vi "Derivative balance.vi"() -> (3 "Motor Power":dbl)   [LabVIEW 2020]
uses:
  Robot Global Data.vi
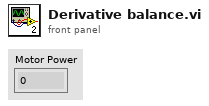
[diagram p1: front panel]
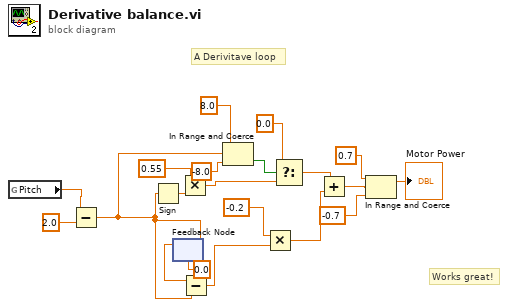
[diagram p0: block diagram]
diagram:
  # "Works great!"
  # "A Derivitave loop"
  n1 = global read "Robot Global Data.vi" "Pitch"() -> (w15:dbl)
  n2 = Subtract(x=w15, y=2.0) -> (x-y=w2:dbl)
  n3 = Sign(1:w2) -> (0:w5:dbl)
  n4 = feedback-in #1(w2) -> ()
  n5 = feedback #1(0.0) -> (w7:dbl)
  n6 = Multiply(x=0.55, y=w5) -> (x*y=w16:dbl)
  n7 = Subtract(x=w7, y=w2) -> (x-y=w19:dbl)
  n8 = In Range and Coerce(upper limit=8.0, x=w2, lower limit=-8.0) -> (In Range?=w12:bool)  [unwired: 1 out]
  n9 = Multiply(x=-0.2, y=w19) -> (x*y=w8:dbl)
  n10 = Select(t=0.0, s=w12, f=w16) -> (s? t:f=w10:dbl)
  n11 = Add(x=w10, y=w8) -> (x+y=w9:dbl)
  n12 = In Range and Coerce(upper limit=0.7, x=w9, lower limit=-0.7) -> (coerced(x)=→"Motor Power":dbl)  [unwired: 1 out]
